vi "Spectrograph_acceptCommand_changeFilter.vi"(8 "error in (no error)":errorcluster, 11 "command_changeFilter_Ctl":T1) -> (0 "error out":errorcluster, 2 "function return":i32, 3 "command_changeFilter_Ctl out":T1)   [LabVIEW 2016, in "SALLV_Spectrograph.lvlib"]
doc: "int Spectrograph_shm_acceptCommand_changeFilterLV(Spectrograph_command_changeFilterLV *command_changeFilter_Ctl );"
uses:
  SALLV_Spectrograph.lvlib
  DataTypes/command_changeFilter.ctl
  SALLV_Spectrograph.so
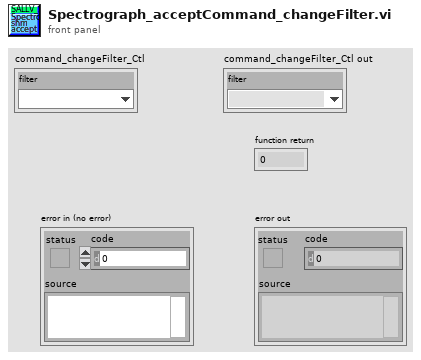
[diagram p1: front panel]
types:
  T1 = typedef "SALLV_Spectrograph.lvlib/command_changeFilter.ctl" = cluster{"filter":enum32{"", "filter0", "filter1", "filter2", "filter3"}}
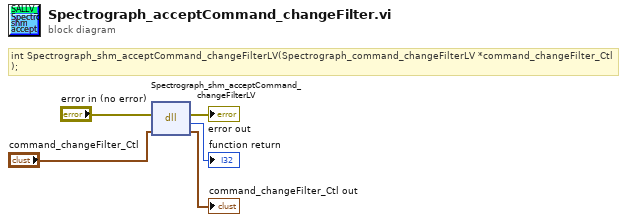
[diagram p0: block diagram]
diagram:
  # "int Spectrograph_shm_acceptCommand_changeFilterLV(Spectrograph_command_changeFilterLV *command_changeFilter_Ctl );"
  n1 = dll-call lib="home/harini/TCS/SALLV_Spectrograph/SALLV_Spectrograph.*" fn="Spectrograph_shm_acceptCommand_changeFilterLV"(error in="error in (no error)", "command_changeFilter_Ctl"="command_changeFilter_Ctl") -> (error out=→"error out":errorcluster, →"function return":i32, "command_changeFilter_Ctl"=→"command_changeFilter_Ctl out":T1)  [unwired: 2 in, 1 out]
